vi "Teleop Arm with Zero Setpoint.vi"(3 "error in (no error)":errorcluster, 4 "Joystick Command":dbl, 5 "MotorControlDevRef":T1) -> (0 "error out":errorcluster, 1 "Commanded\nSet Output":dbl, 2 "MotorControlOutput":T1={"DeviceStatus"={"status"=FALSE, "code"=0, "source"=""}, "Type"=enum."PWM", "PWM"={"PWM Channel"=enum."Invalid", "DeadBand"={"Name"="", "maxPositivePwm"=0, "minPositivePwm"=0, "centerPwm"=0, "maxNegativePwm"=0, "minNegativePwm"=0, "angularRange"=0}}, "CAN"={"Device Number"=0, "SetOutput VI Ref"=variant(refnum<vi> refnum), "GetOutput VI Ref"=variant(refnum<vi> refnum), "Enable VI Ref"=variant(refnum<vi> refnum), "Disable VI Ref"=variant(refnum<vi> refnum), "Data"=variant}, "Invert"=FALSE, "DIO PWM"={"PWM \"Enable\" Channel"=enum."Invalid", "DIOChannel"=enum."Invalid", "PWM Rate"=0.0}})   [LabVIEW 2020]
doc: "This takes a value from a joystick, applies a deadband to the value and then multiples the value by 0.2 to get the value to add to the current setpoint."
uses:
  <vilib>/Rock Robotics/WPI/MotorControl/WPI_MotorControlDeviceRef.ctl
  <vilib>/Rock Robotics/WPI/MotorControl/WPI_MotorControlType.ctl
  <vilib>/Rock Robotics/SystemInterfaces/DIO/FPGA_DIOPWMChannel.ctl
  <vilib>/Rock Robotics/WPI/PWM/WPI_PWMDeadband.ctl
  <vilib>/Rock Robotics/SystemInterfaces/DIO/FPGA_DIOChannel.ctl
  <vilib>/Rock Robotics/WPI/ThirdParty/REV Robotics/REVLib/Typedef/Spark MAX Control Type.ctl
  2022 Robot Global Data.vi
  <vilib>/Rock Robotics/Network Tables/NT Write Number.vi
  2023 Robot Global Data.vi
panel:
  out "Error\n(armSetpoint -\n armPosition)":dbl
  out "Premove\nSensor Position":dbl
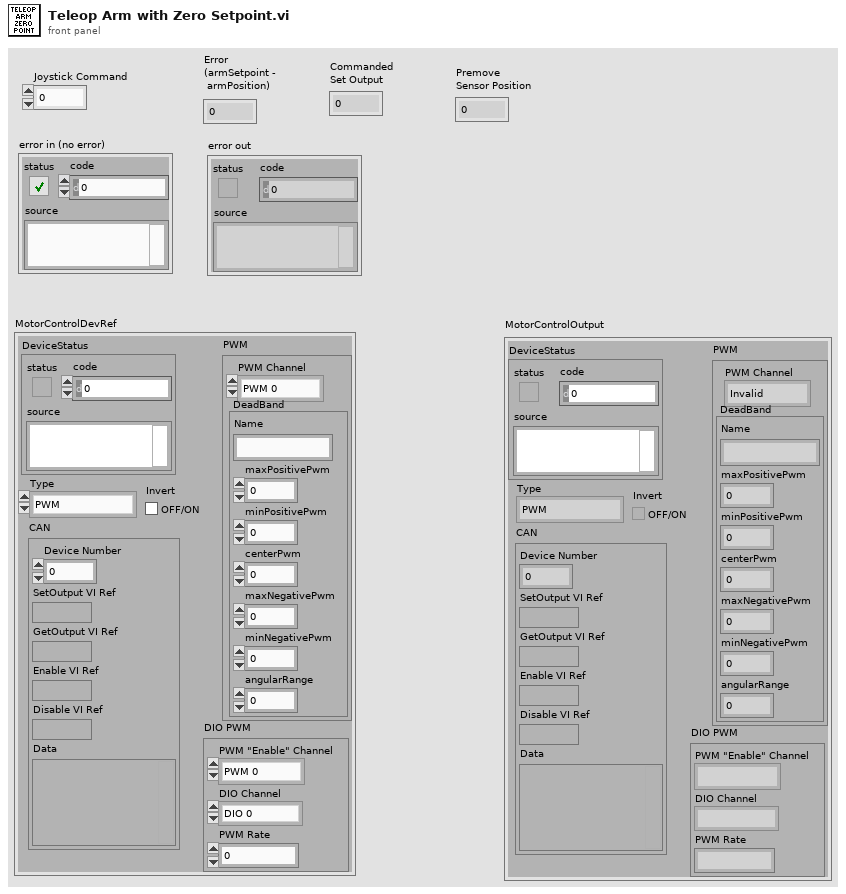
[diagram p1: front panel]
types:
  T1 = typedef "WPI_MotorControlDeviceRef.ctl" = cluster{"DeviceStatus":errorcluster, "Type":T2, "PWM":cluster{"PWM Channel":T3, "DeadBand":T4}, "CAN":cluster{"Device Number":u8, "SetOutput VI Ref":variant, "GetOutput VI Ref":variant, "Enable VI Ref":variant, "Disable VI Ref":variant, "Data":variant}, "Invert":bool, "DIO PWM":cluster{"PWM \"Enable\" Channel":T3, "DIOChannel":T5, "PWM Rate":dbl}}
  T2 = typedef "WPI_MotorControlType.ctl" = enum16{"PWM", "CAN", "DIO PWM"}
  T3 = typedef "FPGA_DIOPWMChannel.ctl" = enum8{"PWM 0", "PWM 1", "PWM 2", "PWM 3", "PWM 4", "PWM 5", "PWM 6", "PWM 7", "PWM 8", "PWM 9", "PWM MXP 0", "PWM MXP 1", "PWM MXP 2", "PWM MXP 3", "PWM MXP 4", "PWM MXP 5", "PWM MXP 6", "PWM MXP 7", "PWM MXP 8", "PWM MXP 9", "Invalid"}
  T4 = typedef "WPI_PWMDeadband.ctl" = cluster{"Name":string, "maxPositivePwm":i32, "minPositivePwm":i32, "centerPwm":i32, "maxNegativePwm":i32, "minNegativePwm":i32, "angularRange":u16}
  T5 = typedef "FPGA_DIOChannel.ctl" = enum8{"DIO 0", "DIO 1", "DIO 2", "DIO 3", "DIO 4", "DIO 5", "DIO 6", "DIO 7", "DIO 8", "DIO 9", "DIO MXP 0", "DIO MXP 1", "DIO MXP 2", "DIO MXP 3", "DIO MXP 4", "DIO MXP 5", "DIO MXP 6", "DIO MXP 7", "DIO MXP 8", "DIO MXP 9", "DIO MXP 10", "DIO MXP 11", "DIO MXP 12", "DIO MXP 13", "DIO MXP 14", "DIO MXP 15", "SPI Port CS1", "SPI Port CS2", "SPI Port CS3", "SPI Port MISO", "SPI Port MOSI", "Invalid"}
  T6 = typedef "Spark MAX Control Type.ctl" = enum16{"Percent VBus", "Voltage", "Velocity", "Position", "Smart Motion", "Current", "Smart Velocity"}
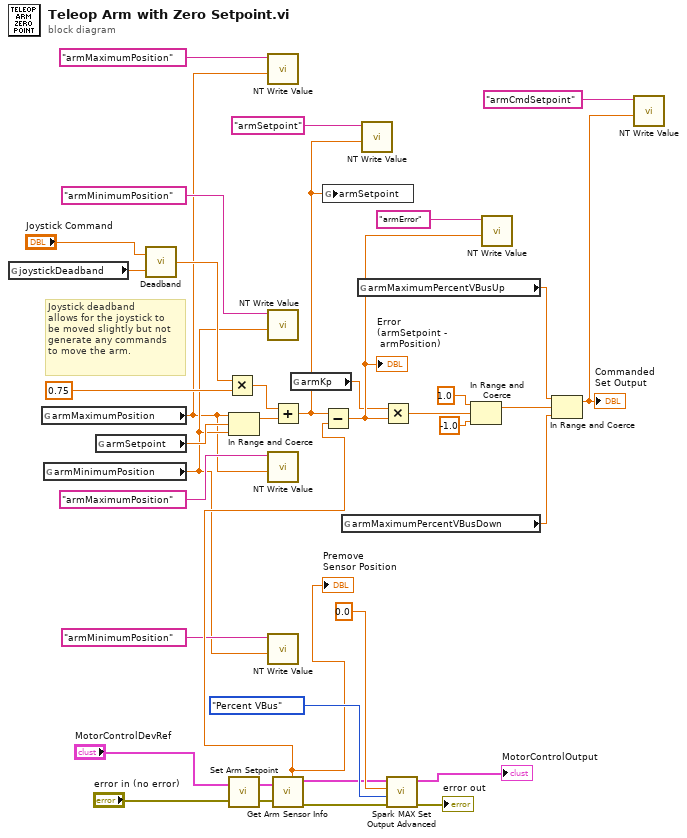
[diagram p0: block diagram]
diagram:
  # "Joystick deadband\nallows for the joystick to\nbe moved slightly but not\ngenerate any commands\nto move the arm."
  n1 = global read "2022 Robot Global Data.vi" "joystickDeadband"() -> (w20:dbl)
  n2 = global read "2022 Robot Global Data.vi" "armMaximumPosition"() -> (w3:dbl)
  n3 = global read "2022 Robot Global Data.vi" "armMinimumPosition"() -> (w5:dbl)
  n4 = global read "2022 Robot Global Data.vi" "armSetpoint"() -> (w26:dbl)
  n5 = call "Deadband.vi"("Limit"=w20, "Input"="Joystick Command") -> ("Output"=w25:dbl)
  n6 = Multiply(x=w25, y=0.75) -> (x*y=w27:dbl)
  n7 = In Range and Coerce(upper limit=w3, x=w26, lower limit=w5) -> (coerced(x)=w28:dbl)  [unwired: 1 out]
  n8 = call "Set Arm Setpoint.vi"("error in (no error)"="error in (no error)", "MotorControlDevRef in"="MotorControlDevRef") -> ("error out"=w19:errorcluster, "MotorControlDevRef out"=w17:T1)
  n9 = call-poly <vilib>:"NT Write Value.vi"("value"=w3, "name"="armMaximumPosition") -> ()  [unwired: 9 in, 1 out]
  n10 = call-poly <vilib>:"NT Write Value.vi"("value"=w5, "name"="armMinimumPosition") -> ()  [unwired: 9 in, 1 out]
  n11 = call-poly <vilib>:"NT Write Value.vi"("value"=w3, "name"="armMaximumPosition") -> ()  [unwired: 9 in, 1 out]
  n12 = call-poly <vilib>:"NT Write Value.vi"("value"=w5, "name"="armMinimumPosition") -> ()  [unwired: 9 in, 1 out]
  n13 = Add(x=w27, y=w28) -> (x+y=w12:dbl)
  n14 = call "Get Arm Sensor Info.vi"("error in (no error)"=w19, "MotorControlDevRef"=w17) -> ("error out"=w16:errorcluster, "MotorControlDevRef out"=w1:T1, "Sensor Position"=w18:dbl)  [unwired: 2 out]
  "Premove\nSensor Position" <- w18
  n15 = global read "2023 Robot Global Data.vi" "armKp"() -> (w2:dbl)
  n16 = global write "2022 Robot Global Data.vi" "armSetpoint"(w12) -> ()
  n17 = Subtract(x=w12, y=w18) -> (x-y=w10:dbl)
  "Error\n(armSetpoint -\n armPosition)" <- w10
  n18 = global read "2022 Robot Global Data.vi" "armMaximumPercentVBusDown"() -> (w21:dbl)
  n19 = global read "2022 Robot Global Data.vi" "armMaximumPercentVBusUp"() -> (w34:dbl)
  n20 = call-poly <vilib>:"NT Write Value.vi"("value"=w12, "name"="armSetpoint") -> ()  [unwired: 9 in, 1 out]
  n21 = Multiply(x=w2, y=w10) -> (x*y=w31:dbl)
  n22 = call <vilib>:"Spark MAX Set Output Advanced.vi"("error in (no error)"=w16, "Control Mode"=Spark_MAX_Control_Type."Percent VBus", "Setpoint"=0.0, "MotorControlDevRef"=w1) -> ("error out"=→"error out":errorcluster, "MotorControlDevRef"=→"MotorControlOutput":T1)  [unwired: 6 in]
  n23 = In Range and Coerce(upper limit=1.0, x=w31, lower limit=-1.0) -> (coerced(x)=w32:dbl)  [unwired: 1 out]
  n24 = call-poly <vilib>:"NT Write Value.vi"("value"=w10, "name"="armError") -> ()  [unwired: 9 in, 1 out]
  n25 = In Range and Coerce(upper limit=w34, x=w32, lower limit=w21) -> (coerced(x)=w14:dbl)  [unwired: 1 out]
  "Commanded\nSet Output" <- w14
  n26 = call-poly <vilib>:"NT Write Value.vi"("value"=w14, "name"="armCmdSetpoint") -> ()  [unwired: 9 in, 1 out]
